vi "LEP_RV_IncBuild_Check.vi"(8 "changed?":bool, 9 "attribute name":string="Target", 10 "default value":refnum<vi>, 11 "control value":variant) -> (0 "changed?":bool, 3 "control value out":variant)   [LabVIEW 2011]
uses:
  <vilib>/Platform/EmbProject/Plugins/utilities/LEP_Utilities_GetSetProjectData_Variant.vi
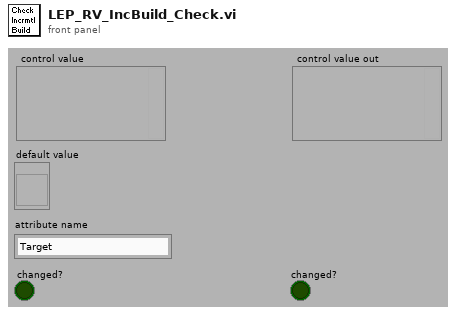
[diagram p1: front panel]
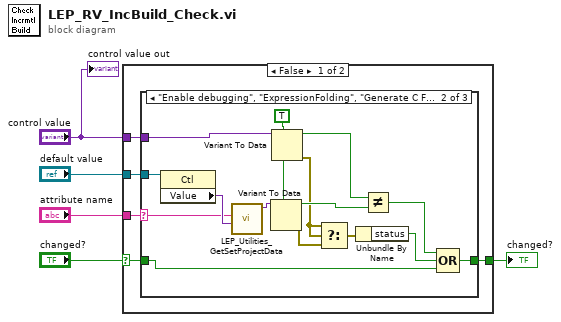
[diagram p0: block diagram]
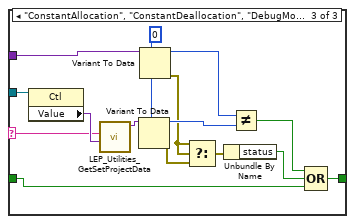
[diagram p3: hidden frame]
diagram:
  n1 = case shown="False" "changed?" {
    selector: "changed?" -> [w6 w42]
    tunnel: "control value" -> [w10 _]
    tunnel: "default value" -> [w9 _]
    tunnel: "attribute name" -> [w8 _]
    tunnel: [w7 w42] -> w4
    frame False {
      n2 = case shown="\"Enable debugging\", \"ExpressionFolding\", \"Generate C Function Calls\", \"GenerateGuardCode\", \"GenerateIntegerOnly\", \"GenerateSerialOnly\", \"UseStackVariables\"" w8 {
        selector: w8 -> [_ w24 w39]
        tunnel: w10 -> [_ w12 w27]
        tunnel: w9 -> [_ w26 w41]
        tunnel: w6 -> [w11 w22 w37]
        tunnel: [w11 w21 w36] -> w7
        frame Default {
        }
        frame "Enable debugging", "ExpressionFolding", "Generate C Function Calls", "GenerateGuardCode", "GenerateIntegerOnly", "GenerateSerialOnly", "UseStackVariables" {
          w18 = TRUE
          n3 = property class="Ctl"(reference=w26) -> ("Value"=w25:variant)  [unwired: 1 in, 2 out]
          n4 = call-poly <vilib>:"LEP_Utilities_GetSetProjectData.vi"("Variant In"=w25, "ItemName"=w24) -> ("Variant Out"=w19:variant)  [unwired: 3 in, 6 out]
          n5 = Variant To Data(type=w18, Variant=w19) -> (data=w16:bool, error out=w14:errorcluster)  [unwired: 1 in]
          n6 = Variant To Data(type=w18, Variant=w12) -> (data=w20:bool, error out=w15:errorcluster)  [unwired: 1 in]
          n7 = Select(t=w15, s=w15, f=w14) -> (s? t:f=w13:errorcluster)
          n8 = Unbundle By Name(w13) -> ("status"=w17:bool)
          n9 = Not Equal?(x=w20, y=w16) -> (x != y?=w23:bool)
          n10 = Compound Arithmetic op=OR(w23, w17, w22) -> (w21:bool)
        }
        frame "ConstantAllocation", "ConstantDeallocation", "DebugMode" {
          w33 = u16 0
          n11 = property class="Ctl"(reference=w41) -> ("Value"=w40:variant)  [unwired: 1 in, 2 out]
          n12 = call-poly <vilib>:"LEP_Utilities_GetSetProjectData.vi"("Variant In"=w40, "ItemName"=w39) -> ("Variant Out"=w34:variant)  [unwired: 3 in, 6 out]
          n13 = Variant To Data(type=w33, Variant=w34) -> (data=w31:u16, error out=w29:errorcluster)  [unwired: 1 in]
          n14 = Variant To Data(type=w33, Variant=w27) -> (data=w35:u16, error out=w30:errorcluster)  [unwired: 1 in]
          n15 = Select(t=w30, s=w30, f=w29) -> (s? t:f=w28:errorcluster)
          n16 = Unbundle By Name(w28) -> ("status"=w32:bool)
          n17 = Not Equal?(x=w35, y=w31) -> (x != y?=w38:bool)
          n18 = Compound Arithmetic op=OR(w38, w32, w37) -> (w36:bool)
        }
      }
    }
    frame True {
    }
  }
  "changed?" <- w4
  "control value out" <- "control value"
